vi "AX_BarCode.vi"() -> ()   [LabVIEW 2011]
panel:
  in  "字符串":string
  in  "BarCodeCtrl":refnum<k7>(container)
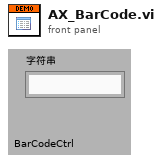
[diagram p1: front panel]
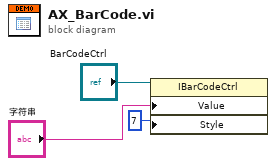
[diagram p0: block diagram]
diagram:
  n1 = property class="IBarCodeCtrl"(reference="BarCodeCtrl", "Value"="字符串", "Style"=i16 7) -> ()  [unwired: 1 in, 2 out]
